vi "ReplaceValArray.vi"(8 "Value":dbl, 9 "y":dbl, 10 "x":dbl, 11 "Array":dbl[](array[numeric])) -> (2 "output array":dbl[](array[numeric]))   [LabVIEW 2017]
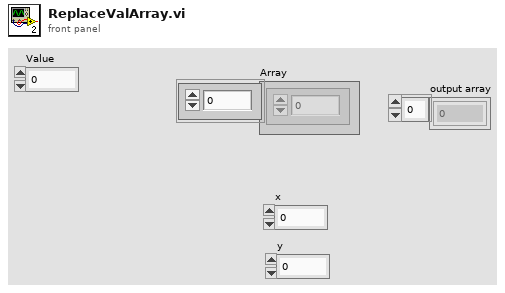
[diagram p1: front panel]
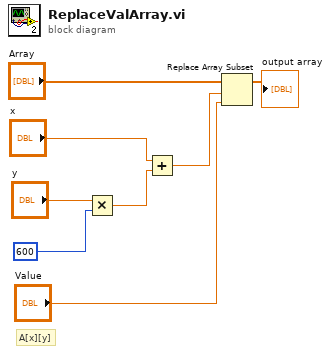
[diagram p0: block diagram]
diagram:
  # "A[x][y]"
  n1 = Multiply(x="y", y=600) -> (x*y=w6:dbl)
  n2 = Add(x="x", y=w6) -> (x+y=w3:dbl)
  n3 = Replace Array Subset(array="Array", new element="Value", index=w3) -> (→"output array":dbl[])
